vi "Test Helper Loop Multiple Parallell Helper Loops.vi"(8 "error in (no error)":errorcluster, 11 "Helper Loop Test In":refnum<class "Helper Loop Test.lvclass">) -> (0 "error out":errorcluster, 3 "Helper Loop Test Out":refnum<class "Helper Loop Test.lvclass">)   [LabVIEW 2020, in "Helper Loop Test.lvclass"]
uses:
  Helper Loop Test.lvclass
  C:/Program Files (x86)/National Instruments/LabVIEW 2020/vi.lib/Astemes/LUnit/Test Case.lvclass
  source/Framework Test Suite/Mock Process/Mock Process.lvclass
  C:/Git/astemes-triarc-framework/source/Framework/Process/Process.lvclass
  source/Framework/Process/Process.lvclass/Process.ctl
  <vilib>/Astemes/LUnit/Test Case.lvclass/Test Case.ctl
  <vilib>/Astemes/LUnit/LUnit Assertion Result.lvclass/LUnit Assertion Result.ctl
  <vilib>/Astemes/LUnit/LUnit Test Case Result.lvclass/LUnit Test Case Result.ctl
  <vilib>/Astemes/LUnit/LUnit Method Result.lvclass/LUnit Method Result.ctl
  50b6e122-0124-4b7b-aa32-eb2a86067106.vi
  42738f38-96e3-4277-8aab-a77fd84bb115.vi
  source/Framework/Process/Public/Lifecycle/Get Lifecycle State.vi
  source/Framework/Broadcast Event Helpers/Execution timer.vi
  <vilib>/Astemes/LUnit/Palette/Pass.vi
  <vilib>/Astemes/LUnit/Palette/Fail.vi
  <vilib>/Astemes/LUnit/Compare Variants.vi
  <vilib>/Astemes/LUnit/Describe Comparison.vi
  <vilib>/Astemes/LUnit/Set Assertion Type.vi
  source/Framework/Process/Private/SubVIs/Wait for finish.vi
  source/Framework/Process/Protected/Messaging/Enqueue Message.vi
  source/Framework/Process/Private/SubVIs/Set Lifecycle State.vi
  <vilib>/Utility/error.llb/Clear Errors.vi
  <vilib>/Astemes/LUnit/Add test result.vi
  <vilib>/Astemes/LUnit/LUnit Write Passed.vi
  <vilib>/Astemes/LUnit/LUnit Write Message.vi
  <vilib>/Astemes/LUnit/LUnit Write Description.vi
  <vilib>/Astemes/LUnit/Variant to string.vi
  <vilib>/Astemes/LUnit/LUnit Write Assertion Type.vi
  source/Framework/Process/Private/SubVIs/Handle Debug Data.vi
  <vilib>/Astemes/LUnit/LUnit Record Assertion Result.vi
  source/Framework/Logging/Log Debug.vi
  <vilib>/AdvancedString/1D String Array to Delimited String.vi
  <vilib>/Utility/High Resolution Relative Seconds.vi
  <vilib>/Astemes/LUnit/LUnit Aggregate Assertion Results.vi
  <vilib>/Astemes/LUnit/Assertion Result/LUnit Read Status.vi
  <vilib>/Astemes/LUnit/LUnit Read Message.vi
  <vilib>/Astemes/LUnit/LUnit Read Description.vi
  <vilib>/Astemes/LUnit/Method Result/LUnit Merge Status.vi
  <vilib>/Astemes/LUnit/LUnit Concatenate result strings.vi
  <vilib>/Utility/error.llb/Error Cluster From Error Code.vi
  source/Framework/Broadcast Event Helpers/Dequeue Broadcast Message.vi
  <vilib>/Utility/Data Type/Get Type Information.vi
  <vilib>/Utility/LVClass/Get LV Class Name.vi
  source/Framework/Process/Public/Read Name.vi
  <vilib>/Astemes/LUnit/LUnit Assertion Result.lvclass
  source/Framework/Process/Process.lvclass
  source/Framework/Broadcast Event Helpers/Broadcast Event Helpers.lvlib
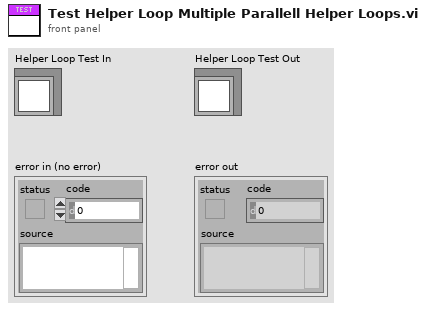
[diagram p1: front panel]
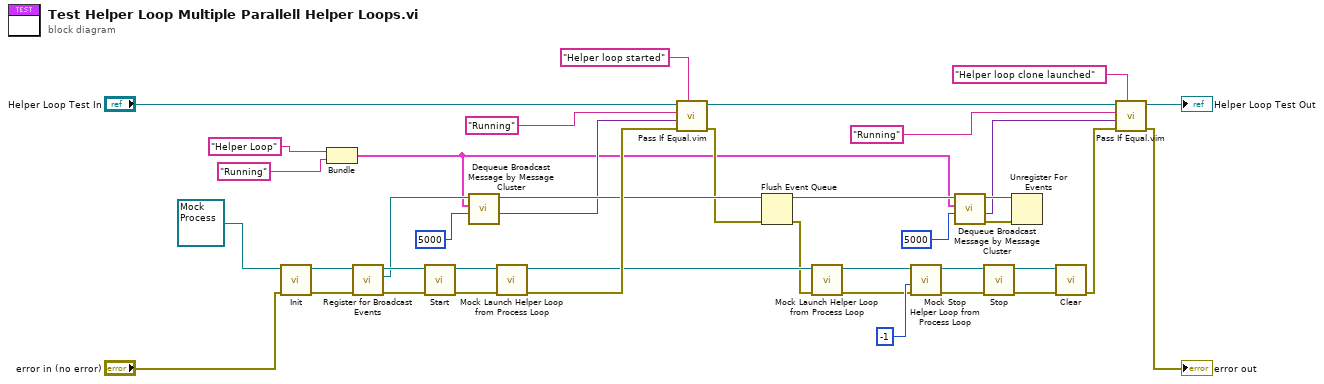
[diagram p0: block diagram]
diagram:
  n1 = call-dynamic "Init.vi"("error in (no error)"="error in (no error)", "Mock Process In"=refnum<class "Mock Process.lvclass"> refnum) -> ("error out"=w40:errorcluster, "Mock Process Out"=w20:refnum<class "Mock Process.lvclass">)  [unwired: 8 in]
  n2 = Bundle("y"="Helper Loop", "Description"="Running") -> (w1:cluster{"y":string, "Description":string})  [unwired: 1 in]
  n3 = call "Register for Broadcast Events.vi"("error in (no error)"=w40, "Process In"=w20) -> ("error out"=w21:errorcluster, "Event Registration Refnum Out"=w16:refnum<event-registration>, "Process Out"=w19:refnum<class "Mock Process.lvclass">)  [unwired: 7 in]
  n4 = call "Start.vi"("error in (no error)"=w21, "Process In"=w19) -> ("error out"=w38:errorcluster, "Process Out"=w39:refnum<class "Mock Process.lvclass">)  [unwired: 7 in, 1 out]
  n5 = call "Dequeue Broadcast Message by Message Cluster.vi"("Timeout (-1)"=5000, "Message"=w1, "Event Registration Refnum"=w16) -> ("Message Data"=w5:variant, "Event Registration Refnum Out"=w13:refnum<event-registration>)  [unwired: 4 in, 3 out]
  n6 = call "Mock Launch Helper Loop from Process Loop.vi"("error in (no error)"=w38, "Mock Process in"=w39) -> ("error out"=w27:errorcluster, "Mock Process out"=w26:refnum<class "Mock Process.lvclass">)  [unwired: 8 in]
  n7 = call "Pass If Equal.vim"("Description"="Helper loop started", "error in (no error)"=w27, "Actual"=w5, "Expected"="Running", "LUnit Test Case In"="Helper Loop Test In") -> ("error out"=w12:errorcluster, "LUnit Test Case Out"=w29:refnum<class "Helper Loop Test.lvclass">)  [unwired: 5 in]
  n8 = Flush Event Queue(0:w13, 3:w12) -> (8:w10:refnum<event-registration>, 11:w11:errorcluster)  [unwired: 4 in, 1 out]
  n9 = call "Mock Launch Helper Loop from Process Loop.vi"("error in (no error)"=w11, "Mock Process in"=w26) -> ("error out"=w17:errorcluster, "Mock Process out"=w18:refnum<class "Mock Process.lvclass">)  [unwired: 8 in]
  n10 = call "Mock Stop Helper Loop from Process Loop.vi"("error in (no error)"=w17, "timeout in ms (-1)"=-1, "Mock Process in"=w18) -> ("error out"=w24:errorcluster, "Mock Process out"=w25:refnum<class "Mock Process.lvclass">)  [unwired: 6 in, 1 out]
  n11 = call "Dequeue Broadcast Message by Message Cluster.vi"("Timeout (-1)"=5000, "Message"=w1, "Event Registration Refnum"=w10) -> ("error out"=w7:errorcluster, "Message Data"=w4:variant, "Event Registration Refnum Out"=w6:refnum<event-registration>)  [unwired: 4 in, 2 out]
  n12 = call "Stop.vi"("error in (no error)"=w24, "Process In"=w25) -> ("error out"=w37:errorcluster, "Process Out"=w22:refnum<class "Mock Process.lvclass">)  [unwired: 7 in, 1 out]
  n13 = Unregister For Events(event registration refnum=w6, error in=w7) -> ()  [unwired: 1 out]
  n14 = call-dynamic "Clear.vi"("error in (no error)"=w37, "Mock Process In"=w22) -> ("error out"=w36:errorcluster)  [unwired: 9 in]
  n15 = call "Pass If Equal.vim"("Description"="Helper loop clone launched", "error in (no error)"=w36, "Actual"=w4, "Expected"="Running", "LUnit Test Case In"=w29) -> ("error out"=→"error out":errorcluster, "LUnit Test Case Out"=→"Helper Loop Test Out":refnum<class "Helper Loop Test.lvclass">)  [unwired: 5 in]
